vi "Verify a VI.vi"(8 "error in":errorcluster, 11 "Test Case In":refnum<class "LUnit Extensions Tests.lvclass">) -> (0 "error out":errorcluster, 3 "Test Case Out":refnum<class "LUnit Extensions Tests.lvclass">)   [LabVIEW 2020, in "LUnit Extensions Tests.lvclass"]
uses:
  Common/Person/Person.lvclass/Person.ctl
  Common/Person/Write First Name.vi
  Common/Person/Write Last Name.vi
  Common/Person/Write Title.vi
  LUnit Extensions Tests.lvclass
  LUnit Extensions Tests.lvclass/LUnit Extensions Tests.ctl
  Source/Extensions/LUnit.Extension/LUnitExtension.lvlib
  C:/Program Files/National Instruments/LabVIEW 2020/vi.lib/Astemes/LUnit/Test Case.lvclass
  C:/Program Files/National Instruments/LabVIEW 2020/vi.lib/Astemes/LUnit/LUnit Runnable.lvclass
  C:/Users/SAS/Desktop/approval-testing/Tests/LUnit.Tests/LUnit Extensions Tests/LUnit Extensions Tests.lvclass
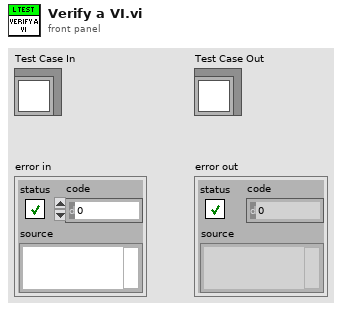
[diagram p1: front panel]
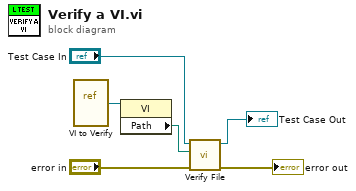
[diagram p0: block diagram]
diagram:
  n1 = vi-ref "VI to Verify.vi"() -> (w2:refnum<vi>)
  n2 = property class="VI"(reference=w2) -> ("Path"=w1:path)  [unwired: 1 in, 2 out]
  n3 = call "Verify File.vi"("error in"="error in", "path to file"=w1, "LUnit Test Case In"="Test Case In") -> ("error out"=→"error out":errorcluster, "LUnit Test Case Out"=→"Test Case Out":refnum<class "LUnit Extensions Tests.lvclass">)  [unwired: 7 in]
